vi "Check If Running.vi"(10 "String":string) -> ()   [LabVIEW 2024, in "Sift Client.lvlib"]
uses:
  Sift Client.lvlib
panel:
  out "error out":errorcluster
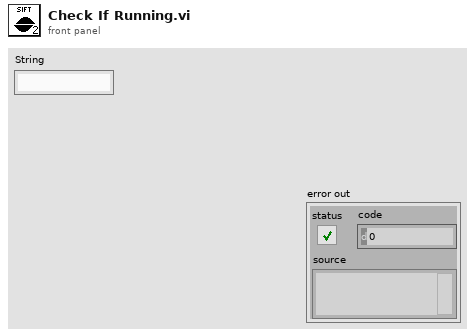
[diagram p1: front panel]
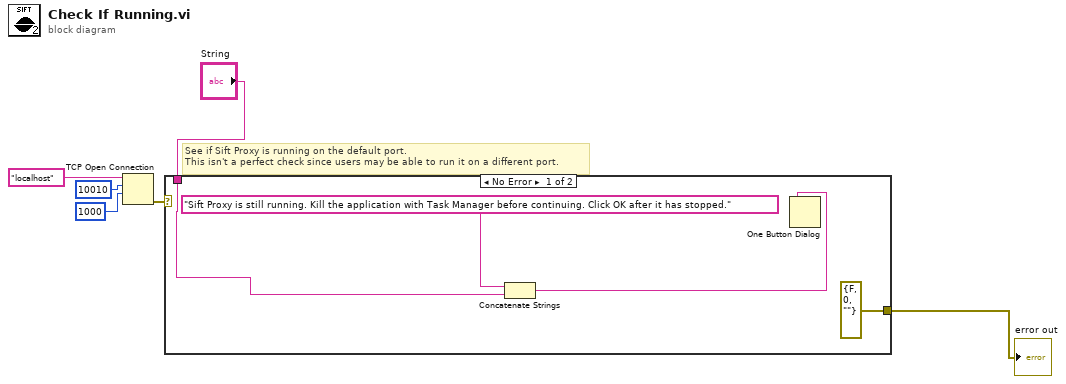
[diagram p0: block diagram]
diagram:
  # "See if Sift Proxy is running on the default port.\nThis isn't a perfect check since users may be able to run it on a different port."
  n1 = TCP Open Connection(address="localhost", remote port or service name=u16 10010, timeout ms (60000)=1000) -> (error out=w3:errorcluster)  [unwired: 2 in, 1 out]
  n2 = case shown="No Error" w3 {
    selector: w3 -> [_ w11]
    tunnel: "String" -> [w9 _]
    tunnel: [errorcluster {"status"=FALSE, "code"=0, "source"=""} ("error out") w11] -> w1
    frame No Error {
      n3 = Concatenate Strings("Sift Proxy is still running. Kill the application with Task Manager before continuing. Click OK after it has stopped." ("message"), w9) -> (w8:string)
      n4 = One Button Dialog(message=w8) -> ()  [unwired: 1 in, 1 out]
    }
    frame Error {
    }
  }
  "error out" <- w1
